vi "PruebaConfigGetSet.vi"   [LabVIEW 2014, in "MSX-E3701.lvlib"]
uses:
  MSX-E3701.lvlib
  MSX-E3701Class/MSX-E3701.lvclass
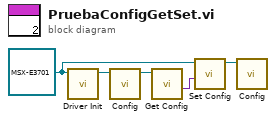
[diagram p0: block diagram]
diagram:
  w1 = refnum<class "MSX-E3701.lvclass"> refnum ("MSX-E3701.lvlib:MSX-E3701.lvclass")
  n1 = call-dynamic "Driver Init.vi"("MSX-E3701 in"=w1) -> ("MSX-E3701 out"=w5:refnum<class "MSX-E3701.lvclass">)  [unwired: 9 in, 1 out]
  n2 = call-dynamic "Config.vi"("MSX-E3701 in"=w5) -> ("MSX-E3701 out"=w4:refnum<class "MSX-E3701.lvclass">)  [unwired: 8 in, 2 out]
  n3 = call-dynamic "Get Config.vi"("MSX-E3701 in"=w4) -> ("Config Data"=w3:variant)  [unwired: 8 in, 2 out]
  n4 = call-dynamic "Set Config.vi"("Variant"=w3, "MSX-E3701 in"=w1) -> ("MSX-E3701 out"=w2:refnum<class "MSX-E3701.lvclass">)  [unwired: 8 in, 1 out]
  n5 = call-dynamic "Config.vi"("MSX-E3701 in"=w2) -> ()  [unwired: 8 in, 3 out]
